vi "FeedbackDecode_20200902.vi"() -> ()   [LabVIEW 2016]
uses:
  FeedbackDecode_DecodeClust.ctl
  FeedbackDecode_MvntClust.ctl
  FeedbackDecode_EncodeClust.ctl
  FeedbackDecode_CogLoadClust.ctl
  <vilib>/Platform/TimedLoop/XDataNode/timing_clust.ctl
  <vilib>/Platform/TimedLoop/XDataNode/nitl_modes.ctl
  <vilib>/Platform/TimedLoop/XDataNode/wakeup.ctl
  <vilib>/DAQmx/write.llb/DAQmx Write (Analog DBL 1Chan 1Samp).vi
  subvi/FeedbackDecode_Globals.vi
  <vilib>/imath/engines/lvmath2/RunTimeEngine/BuiltInFunctions/reshapemx/NIMS_[GM]_reshapemx.vi
  <instcachedir>/0/NIMS_[GM]_reshapemx_500BD31B48F5434EA23B2056DCB44201.lvgen/NIMS_[GM]_reshapemx_500BD31B48F5434EA23B2056DCB44201_005.vi
  <vilib>/imath/engines/lvmath2/RunTimeEngine/BuiltInFunctions/rotate90/NIMS_rotate90.vi
  <instcachedir>/0/NIMS_rotate90_7DC1660D109944E092D2EB6E3185A1B6.lvgen/NIMS_rotate90_7DC1660D109944E092D2EB6E3185A1B6_005.vi
  <vilib>/imath/engines/lvmath2/RunTimeEngine/BuiltInFunctions/reshapemx/NIMS_[GV]_reshapemx.vi
  <instcachedir>/0/NIMS_[GV]_reshapemx_314E456D64644EB191D4916921E89AA6.lvgen/NIMS_[GV]_reshapemx_314E456D64644EB191D4916921E89AA6_001.vi
  <vilib>/imath/engines/lvmath2/RunTimeEngine/ErrorHandling/NIMS_Create Error From Enums.vi
  <vilib>/imath/engines/lvmath2/RunTimeEngine/NodeEndStatement/NIMS_NodeEndStatement_Output.vi
  <instcachedir>/0/NIMS_NodeEndStatement_Output_53EC0D466D134D7ABD903AC30B43404B.lvgen/NIMS_NodeEndStatement_Output_53EC0D466D134D7ABD903AC30B43404B_004.vi
  <vilib>/imath/engines/lvmath2/RunTimeEngine/ErrorHandling/NIMS_Finalize Error.vi
  subvi/FeedbackDecode_VariablesToString_Scalar.vi
  <vilib>/DAQmx/miscellaneous.llb/DAQmx Fill In Error Info.vi
  subvi/FeedbackDecode_VariablesToString_String.vi
  subvi/FeedbackDecode_VariablesToString_Array.vi
  <vilib>/Utility/file.llb/Read Delimited Spreadsheet (string).vi
  <vilib>/Utility/file.llb/Write Delimited Spreadsheet (string).vi
  <vilib>/platform/TimedLoop/XDataNode/XDataNode.xnode
  <vilib>/regexp/Match Regular Expression.xnode
  <vilib>/Platform/TimedLoop/XDataNode/XDNodeRunTimeDep.lvlib
  <resource>/objmgr/daqmx.rc
panel:
  out "CurrMvnt":T1
  in  "Exclude SE":bool
  out "DAQmx?":bool
  out "NumComp":enum16{"1 Computer", "2 Computers"}(ring)
  out "BuildDir":path
  out "PupilTracker":bool
  out "CopySucc":bool
  out "Delete from D drive?":bool
  out "Copy to raid?":bool
  out "Don't save to database?":bool
  out "NextIdx":dbl
  in  "HeatMap Range":cluster{"Min":dbl, "Max":dbl}={"Min"=0.0, "Max"=50.0}
  out "RespRefArray":refnum<vi>[](array[refnum])
  out "VRELabel":T2(ring)
  out "StimTog":bool
  out "SelTog":bool
  out "StimCmd":string
  out "RespStr":string
  out "EvntReg":refnum<event-registration>
  out "MvntEvnt":refnum<user-event>
  out "DataDir":path
  out "PulseStim":bool
  out "BaseCnt3":i64
  out "NIPTime":dbl
  out "ParamsTableLoc":cluster{"Left":i32, "Width":u32}
  out "iTiming":T3
  in  "LVTab":T4(tab)
  out "TrainCnt":dbl
  in  "DecodeClust":T5={"TrainParams"={"Lag"=0.0, "KernelWidth"=0.3, "TargRad"=0.15}, "Kinematics"={"Thumb"=0.0, "Index"=0.0, "Middle"=0.0, "Ring"=0.0, "Little"=0.0, "ThumbInt"=0.0, "IndexInt"=0.0, "RingInt"=0.0, "LittleInt"=0.0, "Wrist"=0.0, "WristYaw"=0.0, "WristRoll"=0.0}, "CtrlButtons"={"AcqTraining"=FALSE, "ApplyBaseline"=FALSE, "ApplyTraining"=FALSE, "LoadTrainFile"=FALSE, "CAR"=FALSE, "NIPSpikes"=FALSE, "AcqBaseline"=FALSE, "Stop"=FALSE, "ResetTrial"=FALSE, "CalDEKA"=FALSE, "HideSphrs"=FALSE, "StartTrials"=FALSE, "AutoPop"=FALSE, "ResetVRE"=FALSE, "StopVRE"=FALSE, "AcqCAR"=FALSE, "ConARD"=FALSE, "DEKARestart"=FALSE, "ConnDEKA"=FALSE}, "CompID"={"LV"={"Name"="PNILABVIEW", "IP"="155.100.90.215"}, "ML"={"Name"="PNIMATLAB", "IP"="155.100.91.231"}}, "KMvntClust"={"KGain"=[[1.0, 1.0, -1.0, 1.0], [1.0, 1.0, -1.0, 1.0], [1.0, 1.0, -1.0, 1.0], [1.0, 1.0, -1.0, 1.0], [1.0, 1.0, -1.0, 1.0], [1.0, 1.0, -1.0, 1.0], [1.0, 1.0, -1.0, 1.0], [1.0, 1.0, -1.0, 1.0], [1.0, 1.0, -1.0, 1.0], [1.0, 1.0, -1.0, 1.0], [1.0, 1.0, -1.0, 1.0], [1.0, 1.0, -1.0, 1.0]], "KMvnts"={"Thumb"=TRUE, "Index"=TRUE, "Middle"=TRUE, "Ring"=TRUE, "Little"=TRUE, "ThumbInt"=TRUE, "IndexInt"=TRUE, "RingInt"=TRUE, "LittleInt"=TRUE, "WristPitch"=TRUE, "WristYaw"=TRUE, "WristRoll"=TRUE}, "KThresh"=[[0.2, 0.2, -1.0, 1.0], [0.2, 0.2, -1.0, 1.0], [0.2, 0.2, -1.0, 1.0], [0.2, 0.2, -1.0, 1.0], [0.2, 0.2, -1.0, 1.0], [0.2, 0.2, -1.0, 1.0], [0.2, 0.2, -1.0, 1.0], [0.2, 0.2, -1.0, 1.0], [0.2, 0.2, -1.0, 1.0], [0.2, 0.2, -1.0, 1.0], [0.2, 0.2, -1.0, 1.0], [0.2, 0.2, -1.0, 1.0]], "CtrlMode"=[enum."Position", enum."Position", enum."Position", enum."Position", enum."Position", enum."Position", enum."Position", enum."Position", enum."Position", enum."Position", enum."Position", enum."Position"], "CtrlSpd"=[1.0, 1.0, 1.0, 1.0, 1.0, 1.0, 1.0, 1.0, 1.0, 1.0, 1.0, 1.0]}, "ClearUEA"=FALSE, "Targets"={"Thumb"=0.0, "Index"=0.0, "Middle"=0.0, "Ring"=0.0, "Little"=0.0, "ThumbInt"=0.0, "IndexInt"=0.0, "RingInt"=0.0, "LittleInt"=0.0, "Wrist"=0.0, "WristYaw"=0.0, "WristRoll"=0.0}, "KUEAArray"=[{"Boolean 1"=FALSE, "Boolean 2"=FALSE, "Boolean 3"=FALSE, "Boolean 4"=FALSE, "Boolean 5"=FALSE, "Boolean 6"=FALSE, "Boolean 7"=FALSE, "Boolean 8"=FALSE, "Boolean 9"=FALSE, "Boolean 10"=FALSE, "Boolean 11"=FALSE, "Boolean 12"=FALSE, "Boolean 13"=FALSE, "Boolean 14"=FALSE, "Boolean 15"=FALSE, "Boolean 16"=FALSE, "Boolean 17"=FALSE, "Boolean 18"=FALSE, "Boolean 19"=FALSE, "Boolean 20"=FALSE, "Boolean 21"=FALSE, "Boolean 22"=FALSE, "Boolean 23"=FALSE, "Boolean 24"=FALSE, "Boolean 25"=FALSE, "Boolean 26"=FALSE, "Boolean 27"=FALSE, "Boolean 28"=FALSE, "Boolean 29"=FALSE, "Boolean 30"=FALSE, "Boolean 31"=FALSE, "Boolean 32"=FALSE, "Boolean 33"=FALSE, "Boolean 34"=FALSE, "Boolean 35"=FALSE, "Boolean 36"=FALSE, "Boolean 37"=FALSE, "Boolean 38"=FALSE, "Boolean 39"=FALSE, "Boolean 40"=FALSE, "Boolean 41"=FALSE, "Boolean 42"=FALSE, "Boolean 43"=FALSE, "Boolean 44"=FALSE, "Boolean 45"=FALSE, "Boolean 46"=FALSE, "Boolean 47"=FALSE, "Boolean 48"=FALSE, "Boolean 49"=FALSE, "Boolean 50"=FALSE, "Boolean 51"=FALSE, "Boolean 52"=FALSE, "Boolean 53"=FALSE, "Boolean 54"=FALSE, "Boolean 55"=FALSE, "Boolean 56"=FALSE, "Boolean 57"=FALSE, "Boolean 58"=FALSE, "Boolean 59"=FALSE, "Boolean 60"=FALSE, "Boolean 61"=FALSE, "Boolean 62"=FALSE, "Boolean 63"=FALSE, "Boolean 64"=FALSE, "Boolean 65"=FALSE, "Boolean 66"=FALSE, "Boolean 67"=FALSE, "Boolean 68"=FALSE, "Boolean 69"=FALSE, "Boolean 70"=FALSE, "Boolean 71"=FALSE, "Boolean 72"=FALSE, "Boolean 73"=FALSE, "Boolean 74"=FALSE, "Boolean 75"=FALSE, "Boolean 76"=FALSE, "Boolean 77"=FALSE, "Boolean 78"=FALSE, "Boolean 79"=FALSE, "Boolean 80"=FALSE, "Boolean 81"=FALSE, "Boolean 82"=FALSE, "Boolean 83"=FALSE, "Boolean 84"=FALSE, "Boolean 85"=FALSE, "Boolean 86"=FALSE, "Boolean 87"=FALSE, "Boolean 88"=FALSE, "Boolean 89"=FALSE, "Boolean 90"=FALSE, "Boolean 91"=FALSE, "Boolean 92"=FALSE, "Boolean 93"=FALSE, "Boolean 94"=FALSE, "Boolean 95"=FALSE, "Boolean 96"=FALSE, "Boolean 97"=FALSE, "Boolean 98"=FALSE, "Boolean 99"=FALSE, "Boolean 100"=FALSE}, {"Boolean 1"=FALSE, "Boolean 2"=FALSE, "Boolean 3"=FALSE, "Boolean 4"=FALSE, "Boolean 5"=FALSE, "Boolean 6"=FALSE, "Boolean 7"=FALSE, "Boolean 8"=FALSE, "Boolean 9"=FALSE, "Boolean 10"=FALSE, "Boolean 11"=FALSE, "Boolean 12"=FALSE, "Boolean 13"=FALSE, "Boolean 14"=FALSE, "Boolean 15"=FALSE, "Boolean 16"=FALSE, "Boolean 17"=FALSE, "Boolean 18"=FALSE, "Boolean 19"=FALSE, "Boolean 20"=FALSE, "Boolean 21"=FALSE, "Boolean 22"=FALSE, "Boolean 23"=FALSE, "Boolean 24"=FALSE, "Boolean 25"=FALSE, "Boolean 26"=FALSE, "Boolean 27"=FALSE, "Boolean 28"=FALSE, "Boolean 29"=FALSE, "Boolean 30"=FALSE, "Boolean 31"=FALSE, "Boolean 32"=FALSE, "Boolean 33"=FALSE, "Boolean 34"=FALSE, "Boolean 35"=FALSE, "Boolean 36"=FALSE, "Boolean 37"=FALSE, "Boolean 38"=FALSE, "Boolean 39"=FALSE, "Boolean 40"=FALSE, "Boolean 41"=FALSE, "Boolean 42"=FALSE, "Boolean 43"=FALSE, "Boolean 44"=FALSE, "Boolean 45"=FALSE, "Boolean 46"=FALSE, "Boolean 47"=FALSE, "Boolean 48"=FALSE, "Boolean 49"=FALSE, "Boolean 50"=FALSE, "Boolean 51"=FALSE, "Boolean 52"=FALSE, "Boolean 53"=FALSE, "Boolean 54"=FALSE, "Boolean 55"=FALSE, "Boolean 56"=FALSE, "Boolean 57"=FALSE, "Boolean 58"=FALSE, "Boolean 59"=FALSE, "Boolean 60"=FALSE, "Boolean 61"=FALSE, "Boolean 62"=FALSE, "Boolean 63"=FALSE, "Boolean 64"=FALSE, "Boolean 65"=FALSE, "Boolean 66"=FALSE, "Boolean 67"=FALSE, "Boolean 68"=FALSE, "Boolean 69"=FALSE, "Boolean 70"=FALSE, "Boolean 71"=FALSE, "Boolean 72"=FALSE, "Boolean 73"=FALSE, "Boolean 74"=FALSE, "Boolean 75"=FALSE, "Boolean 76"=FALSE, "Boolean 77"=FALSE, "Boolean 78"=FALSE, "Boolean 79"=FALSE, "Boolean 80"=FALSE, "Boolean 81"=FALSE, "Boolean 82"=FALSE, "Boolean 83"=FALSE, "Boolean 84"=FALSE, "Boolean 85"=FALSE, "Boolean 86"=FALSE, "Boolean 87"=FALSE, "Boolean 88"=FALSE, "Boolean 89"=FALSE, "Boolean 90"=FALSE, "Boolean 91"=FALSE, "Boolean 92"=FALSE, "Boolean 93"=FALSE, "Boolean 94"=FALSE, "Boolean 95"=FALSE, "Boolean 96"=FALSE, "Boolean 97"=FALSE, "Boolean 98"=FALSE, "Boolean 99"=FALSE, "Boolean 100"=FALSE}], "ReTrain"=FALSE, "TargDist"=[0.0, 0.0, 0.0, 0.0, 0.0, 0.0], "State"=enum."Initialize", "KalmanType"=enum."Mean", "EventStr"="", "SelElect"=1.0, "KinSrc"=enum."Off", "HoverElect"=1.0, "RasterWin"=15.0, "WfCnt"=50.0, "ClearWfs"=FALSE, "ApplyThresh"=FALSE, "ThreshVal"=-5.0, "ThreshMode"=enum."RMS Auto", "DataFolder"="00000000-000000", "ClearEMG"=FALSE, "KEMGClust"={"Boolean 92"=FALSE, "Boolean 82"=FALSE, "Boolean 72"=FALSE, "Boolean 62"=FALSE, "Boolean 52"=FALSE, "Boolean 42"=FALSE, "Boolean 32"=FALSE, "Boolean 22"=FALSE, "Boolean 12"=FALSE, "Boolean 2"=FALSE, "Boolean 93"=FALSE, "Boolean 83"=FALSE, "Boolean 73"=FALSE, "Boolean 63"=FALSE, "Boolean 53"=FALSE, "Boolean 43"=FALSE, "Boolean 33"=FALSE, "Boolean 23"=FALSE, "Boolean 13"=FALSE, "Boolean 3"=FALSE, "Boolean 94"=FALSE, "Boolean 84"=FALSE, "Boolean 74"=FALSE, "Boolean 64"=FALSE, "Boolean 54"=FALSE, "Boolean 44"=FALSE, "Boolean 34"=FALSE, "Boolean 24"=FALSE, "Boolean 14"=FALSE, "Boolean 4"=FALSE, "Boolean 95"=FALSE, "Boolean 85"=FALSE, "Boolean 75"=FALSE, "Boolean 65"=FALSE, "Boolean 55"=FALSE, "Boolean 45"=FALSE, "Boolean 35"=FALSE, "Boolean 25"=FALSE, "Boolean 15"=FALSE, "Boolean 5"=FALSE, "Boolean 96"=FALSE, "Boolean 86"=FALSE, "Boolean 76"=FALSE, "Boolean 66"=FALSE, "Boolean 56"=FALSE, "Boolean 46"=FALSE, "Boolean 36"=FALSE, "Boolean 26"=FALSE, "Boolean 16"=FALSE, "Boolean 6"=FALSE, "Boolean 97"=FALSE, "Boolean 87"=FALSE, "Boolean 77"=FALSE, "Boolean 67"=FALSE, "Boolean 57"=FALSE, "Boolean 47"=FALSE, "Boolean 37"=FALSE, "Boolean 27"=FALSE, "Boolean 17"=FALSE, "Boolean 7"=FALSE, "Boolean 98"=FALSE, "Boolean 88"=FALSE, "Boolean 78"=FALSE, "Boolean 68"=FALSE, "Boolean 58"=FALSE, "Boolean 48"=FALSE, "Boolean 38"=FALSE, "Boolean 28"=FALSE, "Boolean 18"=FALSE, "Boolean 8"=FALSE, "Boolean 99"=FALSE, "Boolean 89"=FALSE, "Boolean 79"=FALSE, "Boolean 69"=FALSE, "Boolean 59"=FALSE, "Boolean 49"=FALSE, "Boolean 39"=FALSE, "Boolean 29"=FALSE, "Boolean 19"=FALSE, "Boolean 9"=FALSE}, "EvntFlag"=FALSE, "FillUEA"=FALSE, "FillEMG"=FALSE, "FillMvnts"=FALSE, "BadUEAElects"=[], "KEMGExtra"=[], "AllPairs"=TRUE, "AutoThresh"=0.4, "BadEMGChans"=[], "LinkedDOF"="{}", "AutoPopType"=enum."Gram", "CARType"=enum."Standard", "*Map"=enum."pNeural/pEMG", "GainFill"=1.0, "ThreshFill"=0.2, "TestType"=enum."MSMS", "Outcome"=enum."---", "TrialCnt"=[[0.0, 0.0, 0.0, 0.0, 0.0, 0.0, 0.0, 0.0, 0.0, 0.0, 0.0, 0.0], [0.0, 0.0, 0.0, 0.0, 0.0, 0.0, 0.0, 0.0, 0.0, 0.0, 0.0, 0.0]], "ClearTrials"=FALSE, "Log10"=FALSE, "KDFFile"="", "LimitExt"=FALSE, "*Prosthesis"=enum."MaleRight", "StartML"=TRUE, "StartMLAux"=TRUE, "StartRec"=TRUE, "DynaThr"=FALSE, "ModeFill"=enum."Position", "SpdFill"=1.0, "DEKAMode"=enum."Position", "FreeParam"=1.0, "GoalNoise"=0.0, "Load NN"=FALSE, "ExportTrain"=FALSE, "NumComp"=enum."2 Computers", "DataDir"="00000000-000000", "BuildDir"="00000000-000000", "LatchingFilter"=FALSE, "Trigger"=FALSE} {"SpdFill" min=0.0 max=10.0 step=0.1; "RasterWin" min=1.0 max=30.0 step=1.0; "ThreshFill" min=0.0 max=10.0 step=0.01; "GainFill" min=0.0 max=10.0 step=0.1; "AutoThresh" min=0.0 max=1.0; "Targets"."LittleInt" min=0.0 max=1.0 step=0.01; "Targets"."WristRoll" min=0.0 max=1.0 step=0.01; "Targets"."WristYaw" min=0.0 max=1.0 step=0.01; "Targets"."Wrist" min=0.0 max=1.0 step=0.01; "Targets"."Little" min=0.0 max=1.0 step=0.01; "Targets"."Thumb" min=0.0 max=1.0 step=0.01; "Targets"."RingInt" min=0.0 max=1.0 step=0.01; "Targets"."IndexInt" min=0.0 max=1.0 step=0.01; "Targets"."ThumbInt" min=0.0 max=1.0 step=0.01; "Targets"."Ring" min=0.0 max=1.0 step=0.01; "Targets"."Middle" min=0.0 max=1.0 step=0.01; "Targets"."Index" min=0.0 max=1.0 step=0.01; "KMvntClust"."CtrlSpd" min=0 max=10; "KMvntClust"."KThresh" min=0 max=1; "KMvntClust"."KGain" min=0; "Kinematics"."LittleInt" min=0.0 max=1.0 step=0.01; "Kinematics"."WristRoll" min=0.0 max=1.0 step=0.01; "Kinematics"."WristYaw" min=0.0 max=1.0 step=0.01; "Kinematics"."Wrist" min=0.0 max=1.0 step=0.01; "Kinematics"."Little" min=0.0 max=1.0 step=0.01; "Kinematics"."Thumb" min=0.0 max=1.0 step=0.01; "Kinematics"."RingInt" min=0.0 max=1.0 step=0.01; "Kinematics"."IndexInt" min=0.0 max=1.0 step=0.01; "Kinematics"."ThumbInt" min=0.0 max=1.0 step=0.01; "Kinematics"."Ring" min=0.0 max=1.0 step=0.01; "Kinematics"."Middle" min=0.0 max=1.0 step=0.01; "Kinematics"."Index" min=0.0 max=1.0 step=0.01; "TrainParams"."TargRad" step=0.05 format="%#.2g"; "TrainParams"."KernelWidth" step=0.05 format="%#.2g"}
  in  "Timing":T3={"Dur"={"ASD"=1000.0, "ARD"=5000.0, "ART"=5000.0, "ETD"=500.0}, "Rnd"={"ASDR"=0.0, "ARDR"=0.0, "ARTR"=0.0, "ETDR"=0.0}, "Act"={"ASDA"=0.0, "ARDA"=0.0, "ARTA"=0.0, "ETDA"=0.0}}
  in  "MvntBuilder":T6={"MvntType"={"Thumb"=enum."False", "Index"=enum."False", "Middle"=enum."False", "Ring"=enum."False", "Little"=enum."False", "ThumbInt"=enum."False", "IndexInt"=enum."False", "RingInt"=enum."False", "LittleInt"=enum."False", "WristPitch"=enum."False", "WristYaw"=enum."False", "WristRoll"=enum."False"}, "MvntParams"={"Amp"=1.0, "Delay"=0.0, "Rise"=0.7, "Hold"=3.0}, "MvntList"=[{"MvntMat"=[[0.0, 0.0, 0.0, 0.0], [0.0, 0.0, 0.0, 0.0], [0.0, 0.0, 0.0, 0.0], [0.0, 0.0, 0.0, 0.0], [0.0, 0.0, 0.0, 0.0], [0.0, 0.0, 0.0, 0.0], [0.0, 0.0, 0.0, 0.0], [0.0, 0.0, 0.0, 0.0], [0.0, 0.0, 0.0, 0.0], [0.0, 0.0, 0.0, 0.0], [0.0, 0.0, 0.0, 0.0], [0.0, 0.0, 0.0, 0.0]], "MvntName"="", "Tracking"=enum."False", "Radius"=0.15}], "Set"=FALSE, "Clear"=FALSE, "Load"=FALSE, "Mode"=enum."Block", "NTrials"=10.0, "TargParams"={"Gain"=1.0, "Radius"=0.15, "Acc"=0.8}, "Save"=FALSE, "PercTrials"=0.0} {"PercTrials" format="%#_2g"; "NTrials" min=1.0 max=100.0 step=1.0; "MvntList"."Radius" min=0.0 max=1.0 step=0.01; "TargParams"."Acc" min=0.0 max=1.0 step=0.01; "TargParams"."Radius" min=0.0 max=1.0 step=0.01; "TargParams"."Gain" min=-1.0 max=1.0 step=0.01; "MvntParams"."Hold" min=0.0 step=0.1; "MvntParams"."Rise" min=0.0 step=0.1; "MvntParams"."Delay" min=0.0 step=0.1; "MvntParams"."Amp" min=-1.0 max=1.0 step=0.1}
  in  "ManualClust":T7 {"WristRoll" scale=-1.0..1.0; "WristYaw" scale=-1.0..1.0; "WristPitch" scale=-1.0..1.0; "LittleInt" scale=-1.0..1.0; "RingInt" scale=-1.0..1.0; "IndexInt" scale=-1.0..1.0; "ThumbInt" scale=-1.0..1.0; "Little" scale=-1.0..1.0; "Ring" scale=-1.0..1.0; "Middle" scale=-1.0..1.0; "Index" scale=-1.0..1.0; "Thumb" scale=-1.0..1.0}
  in  "ManualDOF":T8
  in  "EncodeClust":T9={"ParamsTable"=[], "Sel"=[], "Stim"=FALSE, "StimMode"=enum."Off", "StimStep"=[enum."1uA", enum."1uA", enum."Off"], "Jitter"=FALSE, "Pulse"=FALSE, "BFreq"=0.0, "BAmp"=0.0, "UEAArray"=[{"Boolean 1"=FALSE, "Boolean 2"=FALSE, "Boolean 3"=FALSE, "Boolean 4"=FALSE, "Boolean 5"=FALSE, "Boolean 6"=FALSE, "Boolean 7"=FALSE, "Boolean 8"=FALSE, "Boolean 9"=FALSE, "Boolean 10"=FALSE, "Boolean 11"=FALSE, "Boolean 12"=FALSE, "Boolean 13"=FALSE, "Boolean 14"=FALSE, "Boolean 15"=FALSE, "Boolean 16"=FALSE, "Boolean 17"=FALSE, "Boolean 18"=FALSE, "Boolean 19"=FALSE, "Boolean 20"=FALSE, "Boolean 21"=FALSE, "Boolean 22"=FALSE, "Boolean 23"=FALSE, "Boolean 24"=FALSE, "Boolean 25"=FALSE, "Boolean 26"=FALSE, "Boolean 27"=FALSE, "Boolean 28"=FALSE, "Boolean 29"=FALSE, "Boolean 30"=FALSE, "Boolean 31"=FALSE, "Boolean 32"=FALSE, "Boolean 33"=FALSE, "Boolean 34"=FALSE, "Boolean 35"=FALSE, "Boolean 36"=FALSE, "Boolean 37"=FALSE, "Boolean 38"=FALSE, "Boolean 39"=FALSE, "Boolean 40"=FALSE, "Boolean 41"=FALSE, "Boolean 42"=FALSE, "Boolean 43"=FALSE, "Boolean 44"=FALSE, "Boolean 45"=FALSE, "Boolean 46"=FALSE, "Boolean 47"=FALSE, "Boolean 48"=FALSE, "Boolean 49"=FALSE, "Boolean 50"=FALSE, "Boolean 51"=FALSE, "Boolean 52"=FALSE, "Boolean 53"=FALSE, "Boolean 54"=FALSE, "Boolean 55"=FALSE, "Boolean 56"=FALSE, "Boolean 57"=FALSE, "Boolean 58"=FALSE, "Boolean 59"=FALSE, "Boolean 60"=FALSE, "Boolean 61"=FALSE, "Boolean 62"=FALSE, "Boolean 63"=FALSE, "Boolean 64"=FALSE, "Boolean 65"=FALSE, "Boolean 66"=FALSE, "Boolean 67"=FALSE, "Boolean 68"=FALSE, "Boolean 69"=FALSE, "Boolean 70"=FALSE, "Boolean 71"=FALSE, "Boolean 72"=FALSE, "Boolean 73"=FALSE, "Boolean 74"=FALSE, "Boolean 75"=FALSE, "Boolean 76"=FALSE, "Boolean 77"=FALSE, "Boolean 78"=FALSE, "Boolean 79"=FALSE, "Boolean 80"=FALSE, "Boolean 81"=FALSE, "Boolean 82"=FALSE, "Boolean 83"=FALSE, "Boolean 84"=FALSE, "Boolean 85"=FALSE, "Boolean 86"=FALSE, "Boolean 87"=FALSE, "Boolean 88"=FALSE, "Boolean 89"=FALSE, "Boolean 90"=FALSE, "Boolean 91"=FALSE, "Boolean 92"=FALSE, "Boolean 93"=FALSE, "Boolean 94"=FALSE, "Boolean 95"=FALSE, "Boolean 96"=FALSE, "Boolean 97"=FALSE, "Boolean 98"=FALSE, "Boolean 99"=FALSE, "Boolean 100"=FALSE}, {"Boolean 1"=FALSE, "Boolean 2"=FALSE, "Boolean 3"=FALSE, "Boolean 4"=FALSE, "Boolean 5"=FALSE, "Boolean 6"=FALSE, "Boolean 7"=FALSE, "Boolean 8"=FALSE, "Boolean 9"=FALSE, "Boolean 10"=FALSE, "Boolean 11"=FALSE, "Boolean 12"=FALSE, "Boolean 13"=FALSE, "Boolean 14"=FALSE, "Boolean 15"=FALSE, "Boolean 16"=FALSE, "Boolean 17"=FALSE, "Boolean 18"=FALSE, "Boolean 19"=FALSE, "Boolean 20"=FALSE, "Boolean 21"=FALSE, "Boolean 22"=FALSE, "Boolean 23"=FALSE, "Boolean 24"=FALSE, "Boolean 25"=FALSE, "Boolean 26"=FALSE, "Boolean 27"=FALSE, "Boolean 28"=FALSE, "Boolean 29"=FALSE, "Boolean 30"=FALSE, "Boolean 31"=FALSE, "Boolean 32"=FALSE, "Boolean 33"=FALSE, "Boolean 34"=FALSE, "Boolean 35"=FALSE, "Boolean 36"=FALSE, "Boolean 37"=FALSE, "Boolean 38"=FALSE, "Boolean 39"=FALSE, "Boolean 40"=FALSE, "Boolean 41"=FALSE, "Boolean 42"=FALSE, "Boolean 43"=FALSE, "Boolean 44"=FALSE, "Boolean 45"=FALSE, "Boolean 46"=FALSE, "Boolean 47"=FALSE, "Boolean 48"=FALSE, "Boolean 49"=FALSE, "Boolean 50"=FALSE, "Boolean 51"=FALSE, "Boolean 52"=FALSE, "Boolean 53"=FALSE, "Boolean 54"=FALSE, "Boolean 55"=FALSE, "Boolean 56"=FALSE, "Boolean 57"=FALSE, "Boolean 58"=FALSE, "Boolean 59"=FALSE, "Boolean 60"=FALSE, "Boolean 61"=FALSE, "Boolean 62"=FALSE, "Boolean 63"=FALSE, "Boolean 64"=FALSE, "Boolean 65"=FALSE, "Boolean 66"=FALSE, "Boolean 67"=FALSE, "Boolean 68"=FALSE, "Boolean 69"=FALSE, "Boolean 70"=FALSE, "Boolean 71"=FALSE, "Boolean 72"=FALSE, "Boolean 73"=FALSE, "Boolean 74"=FALSE, "Boolean 75"=FALSE, "Boolean 76"=FALSE, "Boolean 77"=FALSE, "Boolean 78"=FALSE, "Boolean 79"=FALSE, "Boolean 80"=FALSE, "Boolean 81"=FALSE, "Boolean 82"=FALSE, "Boolean 83"=FALSE, "Boolean 84"=FALSE, "Boolean 85"=FALSE, "Boolean 86"=FALSE, "Boolean 87"=FALSE, "Boolean 88"=FALSE, "Boolean 89"=FALSE, "Boolean 90"=FALSE, "Boolean 91"=FALSE, "Boolean 92"=FALSE, "Boolean 93"=FALSE, "Boolean 94"=FALSE, "Boolean 95"=FALSE, "Boolean 96"=FALSE, "Boolean 97"=FALSE, "Boolean 98"=FALSE, "Boolean 99"=FALSE, "Boolean 100"=FALSE}], "AdjClust"={"Add"=FALSE, "Sub"=FALSE, "Val"=[1.0, 100.0, 10.0, 500.0, 0.2], "B"=[FALSE, FALSE, FALSE, FALSE, FALSE], "Inc+"=["x+1", "x+1", "x+10", "x+10", "x+0.1"], "Set"=FALSE, "LoadTable"=FALSE, "SaveTable"=FALSE, "ClearTable"=FALSE, "DeleteSel"=FALSE, "Inc-"=["x-1", "x-1", "x-10", "x-10", "x-0.1"]}, "PresetTable"=[], "SelPreset"=[], "SortClust"={"Region"=FALSE, "Receptor"=FALSE, "Electrode"=FALSE, "Min Amp"=FALSE, "Max Amp"=FALSE, "Min Freq"=FALSE, "Max Freq"=FALSE, "Duration"=FALSE}, "SelSort"={"Sel"=FALSE}, "PresetClust"={"Load"=FALSE, "Clear"=FALSE, "Save"=FALSE, "Del"=FALSE}, "RespClust"={"RespType"=enum."Sensor Map", "OpenResp"=FALSE}, "AmpLimit"=100.0, "FreqLimit"=500.0, "DurLimit"=0.2, "Wait Period"=0.5, "Train Period"=0.5} {"Train Period" min=0.0 max=100.0 step=0.1; "Wait Period" min=0.0 max=100.0 step=0.1; "DurLimit" min=0.0 max=1.0 step=0.01; "FreqLimit" min=0.0 max=500.0 step=1.0; "AmpLimit" min=0.0 max=100.0 step=1.0; "BAmp" min=0.0 max=100.0 step=1.0; "BFreq" min=0.0 max=100.0 step=1.0}
  in  "Sensor Tab Control":enum32{"DEKA", "Analog", "TASKA"}(tab)
  out "DekaSensors":waveform(dbl)[](graph)
  out "StimWfGraph":dbl[](graph)
  in  "Stim Thresholds":dbl[](array[numeric])=[0.0, 0.0, 0.0, 0.0, 0.0, 0.0, 0.0, 0.0, 0.0, 0.0, 0.0, 0.0, 0.0]
  in  "DekaSensorBreakThreshold":dbl[](array[numeric])=[40.0, 40.0, 40.0, 40.0, 40.0, 40.0, 40.0, 40.0, 40.0, 40.0, 40.0, 40.0, 40.0]
  out "AnlgPlot":waveform(dbl)[](graph)=[{"t0"=timestamp(27834 s since 1904-01-01), "dt"=1.0, "Y"=[2.75375102500714]}, {"t0"=timestamp(27834 s since 1904-01-01), "dt"=1.0, "Y"=[2.3160330296785294]}, {"t0"=timestamp(27834 s since 1904-01-01), "dt"=1.0, "Y"=[1.270290647354958]}, {"t0"=timestamp(27834 s since 1904-01-01), "dt"=1.0, "Y"=[1.3014283460420921]}]
  in  "OffSet":dbl
  in  "LoadCyberGlove":bool
  in  "TASKARestPositions":string="Rest Positions"
  in  "ThumbIntSet":dbl caption="ThumbInt" min=0.0 max=1.0
  in  "ThumbSet":dbl caption="Thumb" min=0.0 max=1.0
  in  "PinkySet":dbl caption="Pinky" min=0.0 max=1.0
  in  "RingSet":dbl caption="Ring" min=0.0 max=1.0
  in  "MiddleSet":dbl caption="Middle" min=0.0 max=1.0
  in  "IndexSet":dbl caption="Index" min=0.0 max=1.0
  in  "CalibrateTASKA":bool
  in  "Beta Mode":string(combo)="Fixed"
  in  "Computer Goal":string(combo)="Close"
  out "TASKA Pressure":waveform(dbl)[](graph)=[{"t0"=timestamp(87262 s since 1904-01-01), "dt"=1.0, "Y"=[0.0]}, {"t0"=timestamp(87262 s since 1904-01-01), "dt"=1.0, "Y"=[0.0]}, {"t0"=timestamp(87262 s since 1904-01-01), "dt"=1.0, "Y"=[0.0]}]
  out "TASKA IR":waveform(dbl)[](graph)=[{"t0"=timestamp(87262 s since 1904-01-01), "dt"=1.0, "Y"=[4.0]}, {"t0"=timestamp(87262 s since 1904-01-01), "dt"=1.0, "Y"=[0.0]}, {"t0"=timestamp(87262 s since 1904-01-01), "dt"=1.0, "Y"=[0.0]}]
  in  "TASKA Shared Control":bool
  in  "TASKASharedControlBeta":dbl caption="Beta" min=0.0 max=1.0
  in  "ThumbShare":bool
  in  "IndexShare":bool
  in  "RingShare":bool
  in  "MiddleShare":bool
  in  "Reset Calibration":bool
  in  "TASKASharedControlIncrememnt":dbl caption="Inc." min=0.0 max=1.0
  in  "TASKA Timer":bool
  in  "TASKA Reset Break":bool
  in  "TASKA Reset Success":bool
  out "WAVChart":dbl[](graph)=[0.01885986328125, 0.02471923828125, 0.026458740234375, 0.019622802734375, 0.015625, 0.016571044921875, 0.017852783203125, 0.016937255859375, 0.02349853515625, 0.0262451171875, 0.021697998046875, 0.01995849609375, 0.013427734375, 0.008819580078125, 0.013916015625, 0.016693115234375, 0.0172119140625, 0.023468017578125, 0.0235595703125, 0.018890380859375, 0.022369384765625, 0.022003173828125, 0.019378662109375, 0.017578125, 0.0115966796875, 0.011688232421875, 0.011016845703125, 0.007659912109375, 0.012359619140625, 0.015167236328125, 0.010162353515625, 0.00787353515625, 0.010009765625, 0.01434326171875, 0.018524169921875, 0.019012451171875, 0.019317626953125, 0.019500732421875, 0.021514892578125, 0.021514892578125, 0.0233154296875, 0.02276611328125, 0.0174560546875, 0.018585205078125, 0.019439697265625, 0.01959228515625, 0.0185546875, 0.015594482421875, 0.01593017578125, 0.0162353515625, 0.013427734375, 0.01519775390625, 0.005340576171875, 0.008026123046875, 0.00811767578125, 0.004669189453125, 0.008148193359375, 0.00384521484375, 0.007598876953125, 0.007354736328125, 0.009735107421875, 0.01580810546875, 0.01385498046875, 0.014923095703125, 0.00830078125, 0.005096435546875, 0.008941650390625, 0.01416015625, 0.01220703125, 0.0140380859375, 0.01275634765625, 0.006439208984375, 0.007049560546875, 0.006134033203125, -0.000457763671875, 0.003326416015625, 0.0081787109375, 0.009124755859375, 0.013458251953125, 0.014007568359375, 0.014312744140625, 0.006011962890625, 0.00238037109375, 0.010284423828125, 0.011962890625, 0.009857177734375, 0.00909423828125, 0.016448974609375, 0.01885986328125, 0.01190185546875, 0.010955810546875, 0.01019287109375, 0.00152587890625, 0.00762939453125, 0.008270263671875, 0.00604248046875, 0.010589599609375, 0.0037841796875, 0.0050048828125, 0.007080078125, 0.004669189453125, 0.0064697265625, 0.01068115234375, 0.009521484375, 0.002532958984375, -0.000518798828125, 0.005035400390625, 0.0042724609375, 0.00164794921875, 0.0001220703125, -0.002716064453125, -0.00164794921875, -0.007232666015625, -0.01153564453125, -0.005889892578125, -0.00341796875, -0.008514404296875, -0.007415771484375, -0.00726318359375, -0.007781982421875, -0.009918212890625, -0.010772705078125, -0.00628662109375, -0.001373291015625, -0.0008544921875, -0.003997802734375, 0.003021240234375, 0.003082275390625, 0.000640869140625, 0.00250244140625, 0.002960205078125, 0.00115966796875, 0.000579833984375, -0.002166748046875, -0.00115966796875, -0.006591796875, -0.0128173828125, -0.013275146484375, -0.0157470703125, -0.016204833984375, -0.013885498046875, -0.01531982421875, -0.00897216796875, -0.00762939453125, -0.00738525390625, -0.00311279296875, -0.002166748046875, 0.000244140625, -0.003509521484375, -0.003662109375, 0.001220703125, 0.001251220703125, 0.0001220703125, -0.003692626953125, -0.003997802734375, -0.004364013671875, -9.1552734375e-05, 0.00341796875, 0.000457763671875, -0.000274658203125, -0.0006103515625, 0.00543212890625, 0.001312255859375, 0.003662109375, 0.009765625, 0.004852294921875, 0.003997802734375, 0.00189208984375, -0.000213623046875, -0.006500244140625, -0.006744384765625, -0.0120849609375, -0.012359619140625, -0.003631591796875, -0.005645751953125, -0.0028076171875, 0.00286865234375, -0.00311279296875, -0.005279541015625, 0.001922607421875, -0.003753662109375, -0.000335693359375, -0.00299072265625, 0.001556396484375, 0.00299072265625, 0.006317138671875, 0.006622314453125, -0.003692626953125, -0.007110595703125, 0.001190185546875, -0.002288818359375, 0.00030517578125, 0.007720947265625, 0.003692626953125, 0.006011962890625, 0.007904052734375, 0.0115966796875, 0.01513671875, 0.00421142578125, 0.00299072265625, 0.002532958984375, 0.0009765625, 0.0018310546875, 0.001556396484375, 0.00640869140625, 0.008148193359375, 0.011962890625, 0.01416015625, 0.01055908203125, 0.0126953125, 0.006500244140625, 0.00958251953125, 0.009613037109375, 0.00921630859375, 0.007049560546875, 0.00927734375, 0.011871337890625, 0.015655517578125, 0.0146484375, 0.011627197265625, 0.0162353515625, 0.007965087890625, 0.00146484375, 0.004425048828125, 0.007415771484375, 0.007598876953125, 0.011810302734375, 0.01324462890625, 0.016357421875, 0.0126953125, 0.012451171875, 0.01763916015625, 0.0196533203125, 0.019775390625, 0.021453857421875, 0.025848388671875, 0.023468017578125, 0.01934814453125, 0.019073486328125, 0.020355224609375, 0.021270751953125, 0.024139404296875, 0.02545166015625, 0.0255126953125, 0.027862548828125, 0.027435302734375, 0.030487060546875, 0.029052734375, 0.032196044921875, 0.030120849609375, 0.035552978515625, 0.026611328125, 0.025787353515625, 0.030303955078125, 0.021270751953125, 0.027099609375, 0.032379150390625, 0.03143310546875, 0.02508544921875, 0.03118896484375, 0.029510498046875, 0.0311279296875, 0.03460693359375, 0.0340576171875, 0.027435302734375, 0.03076171875, 0.031707763671875, 0.029815673828125, 0.0341796875, 0.039337158203125, 0.0396728515625, 0.039459228515625, 0.031463623046875, 0.025482177734375, 0.03057861328125, 0.031707763671875, 0.03253173828125, 0.035308837890625, 0.0355224609375, 0.035369873046875, 0.02996826171875, 0.0267333984375, 0.025665283203125, 0.024688720703125, 0.029754638671875, 0.023681640625, 0.02490234375, 0.026458740234375, 0.025726318359375, 0.03436279296875, 0.028411865234375, 0.0225830078125, 0.02349853515625, 0.021270751953125, 0.02691650390625, 0.02520751953125, 0.023101806640625, 0.020782470703125, 0.0198974609375, 0.024200439453125, 0.021148681640625, 0.023406982421875, 0.028289794921875, 0.02862548828125, 0.03240966796875, 0.025634765625, 0.030120849609375, 0.029998779296875, 0.02752685546875, 0.033660888671875, 0.028167724609375, 0.032073974609375, 0.033233642578125, 0.02862548828125, 0.029876708984375, 0.02667236328125, 0.02392578125, 0.02764892578125, 0.026275634765625, 0.023468017578125, 0.031158447265625, 0.0306396484375, 0.022125244140625, 0.022430419921875, 0.025054931640625, 0.02337646484375, 0.025299072265625, 0.02777099609375, 0.03326416015625, 0.02777099609375, 0.025390625, 0.028778076171875, 0.02239990234375, 0.01837158203125, 0.021148681640625, 0.021514892578125, 0.018218994140625, 0.01593017578125, 0.017547607421875, 0.018524169921875, 0.01739501953125, 0.01922607421875, 0.016632080078125, 0.010772705078125, 0.013519287109375, 0.011383056640625, 0.013671875, 0.017242431640625, 0.021636962890625, 0.01922607421875, 0.01593017578125, 0.016571044921875, 0.015777587890625, 0.016693115234375, 0.011260986328125, 0.005828857421875, 0.0068359375, 0.001739501953125, 0.00518798828125, 0.006591796875, 0.00286865234375, 0.015289306640625, 0.011383056640625, 0.01031494140625, 0.00927734375, 0.009307861328125, 0.011199951171875, 0.010894775390625, 0.006927490234375, 0.0115966796875, 0.004638671875, 0.004425048828125, 0.003631591796875, 0.007659912109375, 0.0086669921875, 0.00616455078125, 0.003509521484375, -0.000518798828125, 0.0001220703125, -0.001708984375, -0.0015869140625, 0.002349853515625, 0.0089111328125, 0.007171630859375, 0.0072021484375, 0.004791259765625, 0.00341796875, 0.001068115234375, 0.00341796875, 0.00445556640625, 0.008056640625, 0.009246826171875, 0.011077880859375, 0.006195068359375, 0.005340576171875, 0.00244140625, 0.006561279296875, 0.016021728515625, 0.011322021484375, 0.0079345703125, 0.006622314453125, 0.01080322265625, 0.009796142578125, 0.0028076171875, 0.00439453125, 0.00048828125, 0.0052490234375, 0.0025634765625, 0.00396728515625, 0.0057373046875, 0.00860595703125, 0.00701904296875, 0.0020751953125, -0.00189208984375, -0.001861572265625, 0.00091552734375, -0.00762939453125, -0.0074462890625, -0.0054931640625, 0.0010986328125, 0.00421142578125, 0.001800537109375, 0.007232666015625, -0.001190185546875, 9.1552734375e-05, -0.0078125, -0.010833740234375, -0.0068359375, -0.0054931640625, -0.004791259765625, -0.011016845703125, -0.009765625, -0.007720947265625, -0.00384521484375, -0.011260986328125, -0.00848388671875, -0.000152587890625, -0.00030517578125, -0.00177001953125, -0.0052490234375, -0.00994873046875, -0.001617431640625, -0.00567626953125, -0.008209228515625, -0.004638671875, -0.0057373046875, -0.0067138671875, -0.01080322265625, -0.008544921875, -0.0120849609375, -0.009857177734375, -0.01409912109375, -0.0184326171875, -0.022003173828125, -0.023101806640625, -0.02197265625, -0.021942138671875, -0.018035888671875, -0.016632080078125, -0.025726318359375, -0.032623291015625, -0.02557373046875, -0.03179931640625, -0.020660400390625, -0.017578125, -0.01641845703125, -0.017852783203125, -0.02423095703125, -0.030609130859375, -0.03009033203125, -0.027862548828125, -0.031646728515625, -0.03076171875, -0.0225830078125, -0.015472412109375, -0.018341064453125, -0.02520751953125, -0.032958984375, -0.034759521484375, -0.034637451171875, -0.033233642578125, -0.031768798828125, -0.025238037109375, -0.02752685546875, -0.03057861328125, -0.0286865234375, -0.03204345703125, -0.02850341796875, -0.020965576171875, -0.022735595703125, -0.02435302734375, -0.024383544921875, -0.02496337890625, -0.01910400390625, -0.0230712890625, -0.0225830078125, -0.02435302734375, -0.027984619140625, -0.027740478515625, -0.026153564453125, -0.03021240234375, -0.030792236328125, -0.0277099609375, -0.0250244140625, -0.02239990234375, -0.025146484375, -0.029571533203125, -0.022491455078125, -0.02587890625, -0.02081298828125, -0.024688720703125, -0.026885986328125, -0.026214599609375, -0.025482177734375, -0.027374267578125, -0.03387451171875, -0.03570556640625, -0.0379638671875, -0.03662109375, -0.034637451171875, -0.03826904296875, -0.0408935546875, -0.037384033203125, -0.038177490234375, -0.039337158203125, -0.03564453125, -0.02972412109375, -0.02410888671875, -0.01873779296875, -0.02288818359375, -0.02679443359375, -0.03839111328125, -0.0316162109375, -0.029449462890625, -0.02972412109375, -0.03564453125, -0.034332275390625, -0.038665771484375, -0.044525146484375, -0.040374755859375, -0.039031982421875, -0.03741455078125, -0.039703369140625, -0.0386962890625, -0.036834716796875, -0.03521728515625, -0.033905029296875, -0.02984619140625, -0.035430908203125, -0.032440185546875, -0.029022216796875, -0.024688720703125, -0.024139404296875, -0.027099609375, -0.027313232421875, -0.02496337890625, -0.02203369140625, -0.0244140625, -0.021240234375, -0.02392578125, -0.020782470703125, -0.01873779296875, -0.0208740234375, -0.0208740234375, -0.022491455078125, -0.01806640625, -0.0216064453125, -0.017181396484375, -0.01397705078125, -0.01556396484375, -0.009979248046875, -0.016693115234375, -0.01068115234375, -0.016754150390625, -0.01959228515625, -0.016143798828125, -0.02447509765625, -0.029266357421875, -0.026947021484375, -0.02496337890625, -0.0345458984375, -0.027618408203125, -0.0318603515625, -0.028656005859375, -0.02685546875, -0.025634765625, -0.02392578125, -0.026031494140625, -0.014617919921875, -0.018585205078125, -0.021697998046875, -0.019317626953125, -0.02044677734375, -0.0184326171875, -0.018951416015625, -0.022125244140625, -0.019073486328125, -0.02203369140625, -0.0224609375, -0.02166748046875, -0.019073486328125, -0.015411376953125, -0.016448974609375, -0.023834228515625, -0.021728515625, -0.016387939453125, -0.009490966796875, -0.012542724609375, -0.0169677734375, -0.017822265625, -0.02105712890625, -0.017913818359375, -0.016815185546875, -0.01983642578125, -0.0179443359375, -0.0123291015625, -0.01129150390625, -0.01324462890625, -0.015869140625, -0.01385498046875, -0.016387939453125, -0.015655517578125, -0.0181884765625, -0.017578125, -0.013092041015625, -0.008331298828125, -0.007781982421875, -0.00439453125, -0.007080078125, -0.010223388671875, -0.01239013671875, -0.014923095703125, -0.01080322265625, -0.001983642578125, -0.0074462890625, -0.017791748046875, -0.023040771484375, -0.02978515625, -0.0267333984375, -0.0224609375, -0.017120361328125, -0.024871826171875, -0.01788330078125, -0.012298583984375, -0.011566162109375, -0.00726318359375, -0.00457763671875, -0.00299072265625, 0.00146484375, -0.0037841796875, -0.008819580078125, -0.0076904296875, -0.006256103515625, 0.001373291015625, -0.001708984375, -0.00335693359375, 0.001953125, 0.005859375, 0.00396728515625, 0.007110595703125, 0.011993408203125, 0.005828857421875, 0.00677490234375, 0.000244140625, 0.008575439453125, 0.0098876953125, 0.003875732421875, 0.0067138671875, 0.000946044921875, 0.00274658203125, 0.001800537109375, 0.00506591796875, 0.006072998046875, -0.006103515625, -0.00909423828125, -0.003936767578125, -0.001861572265625, -0.002777099609375, 0.001495361328125, 0.0006103515625, -0.003265380859375, -0.0003662109375, 0.00128173828125, 0.0010986328125, 0.002655029296875, -0.005615234375, -0.01275634765625, -0.00775146484375, -0.004913330078125, -0.004119873046875, -0.00506591796875, -9.1552734375e-05, 0.003204345703125, -0.002410888671875, -0.001800537109375, 0.001312255859375, 0.003173828125, -0.002899169921875, -0.004608154296875, 0.002593994140625, -0.002685546875, -0.00762939453125, -0.0028076171875, -0.006805419921875, -0.0146484375, -0.009979248046875, -0.00177001953125, 0.00286865234375, -0.0091552734375, -0.01495361328125, -0.01080322265625, -0.009368896484375, 0.0023193359375, -0.0010986328125, -0.001678466796875, -0.00177001953125, -0.006134033203125, -0.004730224609375, -0.00921630859375, -0.00909423828125, -0.0108642578125, -0.017181396484375, -0.015289306640625, -0.01458740234375, -0.013336181640625, -0.0057373046875, -0.004852294921875, -0.005645751953125, -0.0050048828125, -0.006500244140625, -0.00927734375, -0.012908935546875, -0.014404296875, -0.0155029296875, -0.0115966796875, -0.009796142578125, -0.01202392578125, -0.018157958984375, -0.021240234375, -0.015533447265625, -0.01629638671875, -0.01318359375, -0.015594482421875, -0.020721435546875, -0.017974853515625, -0.02056884765625, -0.02264404296875, -0.01654052734375, -0.01702880859375, -0.0146484375, -0.013275146484375, -0.023040771484375, -0.015960693359375, -0.013092041015625, -0.011077880859375, -0.009063720703125, -0.01727294921875, -0.018035888671875, -0.01580810546875, -0.011932373046875, -0.01287841796875, -0.003692626953125, -0.015167236328125, -0.014068603515625, -0.01666259765625, -0.0211181640625, -0.01812744140625, -0.013336181640625, -0.01519775390625, -0.0093994140625, -0.012847900390625, -0.0208740234375, -0.01300048828125, -0.006988525390625, -0.006072998046875, -0.011199951171875, -0.01263427734375, -0.01263427734375, -0.015625, -0.01055908203125, -0.00372314453125, -0.001312255859375, 0.001861572265625, -6.103515625e-05, -0.00311279296875, -0.001251220703125, -0.006500244140625, -0.00665283203125, 0.000823974609375, 0.001190185546875, 0.004486083984375, -0.004638671875, -0.00250244140625, -0.000518798828125, 0.001739501953125, 0.010955810546875, 0.00384521484375, -0.002349853515625, -0.00128173828125, -0.002227783203125, -0.005157470703125, -0.003204345703125, -0.00482177734375, -0.006072998046875, -0.001312255859375, -0.00018310546875, 0.0001220703125, -0.000274658203125, 0.003753662109375, 0.0103759765625, 0.009063720703125, 0.01324462890625, 0.019989013671875, 0.01324462890625, 0.015350341796875, 0.017791748046875, 0.019744873046875, 0.0157470703125, 0.007049560546875, 0.01263427734375, 0.0111083984375, 0.009002685546875, 0.01141357421875, 0.016632080078125, 0.012847900390625, 0.007568359375, 0.0042724609375, -0.00372314453125, -0.011383056640625, 0.00128173828125, 0.014312744140625, 0.016082763671875, 0.021697998046875, 0.020172119140625, 0.021575927734375, 0.02032470703125, 0.02215576171875, 0.02471923828125, 0.0302734375, 0.02752685546875, 0.02667236328125, 0.026580810546875, 0.0250244140625, 0.027557373046875, 0.020172119140625, 0.0247802734375, 0.02978515625, 0.030120849609375, 0.03131103515625, 0.031524658203125, 0.032257080078125, 0.0286865234375, 0.03033447265625, 0.0279541015625, 0.03582763671875, 0.036285400390625, 0.03515625, 0.028656005859375, 0.0311279296875, 0.033599853515625, 0.03582763671875, 0.028839111328125, 0.02947998046875, 0.0306396484375, 0.025146484375, 0.020843505859375, 0.027679443359375, 0.028045654296875, 0.02532958984375, 0.024017333984375, 0.02410888671875, 0.032073974609375, 0.018951416015625, 0.02801513671875, 0.0318603515625, 0.02587890625, 0.02825927734375, 0.025421142578125, 0.033203125, 0.03515625, 0.0362548828125, 0.030975341796875, 0.034332275390625, 0.02392578125, 0.027191162109375, 0.03472900390625, 0.03515625, 0.02813720703125, 0.0291748046875, 0.028717041015625, 0.027099609375, 0.02874755859375, 0.02203369140625, 0.019805908203125, 0.0179443359375, 0.0289306640625, 0.023773193359375, 0.017059326171875, 0.020904541015625, 0.0262451171875, 0.022979736328125, 0.021453857421875, 0.024017333984375, 0.02056884765625, 0.022430419921875, 0.02081298828125, 0.021759033203125, 0.026611328125, 0.033660888671875, 0.027374267578125, 0.02435302734375, 0.0185546875, 0.018096923828125, 0.023223876953125, 0.01654052734375, 0.015899658203125, 0.009490966796875, 0.00897216796875, 0.00933837890625, 0.013763427734375, 0.01470947265625, 0.021392822265625, 0.0238037109375, 0.022979736328125, 0.025665283203125, 0.0169677734375, 0.0174560546875, 0.015472412109375, 0.012786865234375, 0.011688232421875, 0.0103759765625, 0.00640869140625, 0.0113525390625, 0.0142822265625, 0.012603759765625, 0.0142822265625, 0.016815185546875, 0.020782470703125, 0.012237548828125, 0.008392333984375, 0.017578125, 0.019775390625, 0.026336669921875, 0.02557373046875, 0.019317626953125, 0.015380859375, 0.0196533203125, 0.01812744140625, 0.020050048828125, 0.015045166015625, 0.01416015625, 0.01129150390625, 0.00885009765625, 0.00799560546875, 0.01055908203125, 0.0107421875, 0.0164794921875, 0.0133056640625, 0.0064697265625, 0.0089111328125, 0.0069580078125, 0.0064697265625, 0.001220703125, -0.003082275390625, -0.0028076171875, -9.1552734375e-05, 0.00201416015625, -0.000946044921875, -0.001495361328125, 0.000579833984375, 0.003265380859375, 0.00390625, 0.005889892578125, 0.002685546875, -0.000732421875, 0.004058837890625, 0.0023193359375, 0.008544921875, 0.00250244140625, -0.000885009765625, -0.00244140625, -0.004608154296875, -0.002288818359375, -0.0050048828125, -0.000885009765625, -0.0013427734375, 0.001800537109375, 0.001678466796875, -0.005279541015625, 0.00506591796875, 0.002899169921875, 0.003662109375, 0.0087890625, 0.011474609375, 0.01422119140625, 0.01055908203125, 0.011444091796875, 0.012359619140625, 0.001190185546875, 0.0054931640625, 0.007598876953125, 0.01025390625, 0.01300048828125, 0.008575439453125, 0.007659912109375, 0.00897216796875, 0.014892578125, 0.01226806640625, 0.014434814453125, 0.022003173828125, 0.02056884765625, 0.022705078125, 0.02532958984375, 0.02154541015625, 0.02130126953125, 0.01788330078125, 0.016845703125, 0.018524169921875, 0.015167236328125, 0.01947021484375, 0.017578125, 0.01470947265625, 0.015533447265625, 0.015594482421875, 0.00836181640625, 0.0164794921875, 0.017608642578125, 0.012481689453125, 0.01287841796875, 0.01123046875, 0.010986328125, 0.01324462890625, 0.015655517578125, 0.01287841796875, 0.0107421875, 0.012908935546875, 0.00885009765625, 0.00201416015625, 0.008026123046875, 0.00994873046875, 0.011444091796875, 0.010894775390625, 0.01385498046875, 0.0174560546875, 0.014495849609375, 0.009246826171875, 0.00982666015625, 0.010406494140625, 0.015411376953125, 0.01507568359375, 0.0067138671875, 0.009521484375, 0.011322021484375, 0.00811767578125, -0.002410888671875, 0.00299072265625, -0.004852294921875, 0.0032958984375, 0.0032958984375, 6.103515625e-05, 0.00152587890625, 0.003082275390625, 0.011627197265625, 0.013458251953125, 0.01239013671875, 0.015777587890625, 0.023406982421875, 0.027923583984375, 0.024139404296875, 0.020721435546875, 0.022308349609375, 0.026519775390625, 0.019256591796875, 0.013214111328125, 0.0146484375, 0.015777587890625, 0.02001953125, 0.0150146484375, 0.01055908203125, 0.00897216796875, 0.00823974609375, 0.0013427734375, 0.005615234375, -0.00225830078125, -0.008087158203125, 0.005950927734375, 0.00762939453125, 0.003326416015625, 0.009002685546875, 0.006744384765625, 0.0101318359375, 0.00732421875, 0.004425048828125, 0.01068115234375, 0.001251220703125, 0.008758544921875, 0.018218994140625, 0.013885498046875, 0.014617919921875, 0.011383056640625, 0.01373291015625, 0.0115966796875, 0.00567626953125, 0.002716064453125, -0.000823974609375, 0.0025634765625, 0.0028076171875, 0.002044677734375, -0.000335693359375, 0.0029296875, 0.002655029296875, 0.002349853515625, 0.001678466796875, 0.00433349609375, 0.011871337890625, 0.006744384765625, 0.001129150390625, 0.000640869140625, -0.00042724609375, -0.007781982421875, -0.00433349609375, -0.002166748046875, 0.00189208984375, 0.000823974609375, -0.001922607421875, -0.000152587890625, -0.001007080078125, -0.005035400390625, -0.006439208984375, -0.00799560546875, -0.0150146484375, -0.017822265625, -0.02020263671875, -0.012542724609375, -0.01116943359375, -0.012298583984375, -0.017974853515625, -0.011810302734375, -0.009674072265625, -0.01446533203125, -0.0096435546875, -0.017852783203125, -0.0228271484375, -0.024505615234375, -0.022064208984375, -0.01568603515625, -0.01495361328125, -0.017242431640625, -0.014862060546875, -0.011871337890625, -0.009979248046875, -0.007965087890625, -0.007598876953125, -0.00628662109375, -0.009613037109375, -0.00982666015625, -0.0140380859375, -0.013275146484375, -0.016510009765625, -0.02313232421875, -0.019744873046875, -0.02117919921875, -0.024261474609375, -0.023406982421875, -0.025634765625, -0.026123046875, -0.029937744140625, -0.0272216796875, -0.025054931640625, -0.0198974609375, -0.020263671875, -0.022705078125, -0.0177001953125, -0.018585205078125, -0.020751953125, -0.01678466796875, -0.017181396484375, -0.016937255859375, -0.01995849609375, -0.014312744140625, -0.015350341796875, -0.016815185546875, -0.014129638671875, -0.02496337890625, -0.019317626953125, -0.023193359375, -0.017059326171875, -0.015533447265625, -0.020843505859375, -0.01788330078125, -0.021575927734375, -0.016876220703125, -0.0162353515625, -0.01556396484375, -0.02313232421875, -0.017822265625, -0.011871337890625, -0.0125732421875, -0.01348876953125, -0.014312744140625, -0.00909423828125, -0.009063720703125, -0.010345458984375, -0.00726318359375, -0.01397705078125, -0.009490966796875, -0.00982666015625, -0.007598876953125, -0.00421142578125, -0.00067138671875, 0.001953125, 0.001556396484375, 0.001220703125, -0.009185791015625, -0.013336181640625, -0.01556396484375, -0.01116943359375, -0.0096435546875, -0.010162353515625, -0.011749267578125, -0.012359619140625, -0.009124755859375, -0.009857177734375, -0.011474609375, -0.007568359375, -0.0068359375, -0.0062255859375, -0.00482177734375, -0.010467529296875, -0.0078125, -0.00750732421875, -0.01434326171875, -0.01361083984375, -0.0181884765625, -0.020782470703125, -0.007568359375, -0.006988525390625, -0.006622314453125, -0.001861572265625, -0.00128173828125, -0.0115966796875, -0.005401611328125, -0.004974365234375, -0.0084228515625, -0.011383056640625, -0.0118408203125, -0.008148193359375, -0.006256103515625, -0.001861572265625, 0.004302978515625, 0.004913330078125, 0.006195068359375, 0.00897216796875, 0.003753662109375, 0.00360107421875, -0.00201416015625, -0.001190185546875, -0.0030517578125, -0.0067138671875, -0.00469970703125, -0.005828857421875, -0.005645751953125, 0.001708984375, 0.002960205078125, 0.005767822265625, 0.001983642578125, 0.00048828125, -0.00103759765625, -0.001556396484375, 0.0, 0.007659912109375, 0.01202392578125, 0.010986328125, 0.0059814453125, 0.007354736328125, 0.01275634765625, 0.010009765625, 0.008880615234375, 0.008544921875, 0.007354736328125, 0.001800537109375, 0.00115966796875, -0.002410888671875, 0.009063720703125, 0.01190185546875, 0.012908935546875, 0.010650634765625, 0.004974365234375, 0.01251220703125, 0.012603759765625, 0.007110595703125, 0.00860595703125, 0.017303466796875, 0.01348876953125, 0.01556396484375, 0.0159912109375, 0.0147705078125, 0.01861572265625, 0.014068603515625, 0.0167236328125, 0.015533447265625, 0.0198974609375, 0.019866943359375, 0.015350341796875, 0.0079345703125, 0.0091552734375, 0.00921630859375, 0.011077880859375, 0.00738525390625, 0.008544921875, 0.01690673828125, 0.01513671875, 0.010009765625, 0.0107421875, 0.009674072265625, 0.0142822265625, 0.015899658203125, 0.012359619140625, 0.0203857421875, 0.02166748046875, 0.02032470703125, 0.02069091796875, 0.018280029296875, 0.010772705078125, 0.0057373046875, 0.013519287109375, 0.017242431640625, 0.011383056640625, 0.0142822265625, 0.013824462890625, 0.011962890625, 0.010284423828125, 0.0089111328125, 0.011993408203125, 0.0103759765625, -3.0517578125e-05, -0.00640869140625, -0.00506591796875, -0.00701904296875, -0.003143310546875, 0.0037841796875, 0.008209228515625, 0.00518798828125, 0.00506591796875, 0.006591796875, 0.00701904296875, 0.00567626953125, 0.011383056640625, 0.00543212890625, 0.001556396484375, 0.009185791015625, 0.00628662109375, 0.009521484375, 0.01324462890625, 0.0198974609375, 0.01837158203125, 0.017669677734375, 0.0103759765625, 0.013214111328125, 0.015594482421875, 0.014495849609375, 0.013092041015625, 0.010711669921875, 0.006195068359375, 0.0054931640625, 0.012969970703125, 0.01123046875, 0.017974853515625, 0.015106201171875, 0.011505126953125, 0.009307861328125, 0.024322509765625, 0.023284912109375, 0.01983642578125, 0.025726318359375, 0.030059814453125, 0.0242919921875, 0.02655029296875, 0.03326416015625, 0.023712158203125, 0.02374267578125, 0.022552490234375, 0.0157470703125, 0.020782470703125, 0.022064208984375, 0.022430419921875, 0.0272216796875, 0.02301025390625, 0.019744873046875, 0.018768310546875, 0.0240478515625, 0.029876708984375, 0.032196044921875, 0.030975341796875, 0.026458740234375, 0.025421142578125, 0.023529052734375, 0.024505615234375, 0.021697998046875, 0.018768310546875, 0.0145263671875, 0.01544189453125, 0.0244140625, 0.0198974609375, 0.017578125, 0.021148681640625, 0.01885986328125, 0.0191650390625, 0.018890380859375, 0.02740478515625, 0.018646240234375, 0.02069091796875, 0.025787353515625, 0.02423095703125, 0.0245361328125, 0.022796630859375, 0.01898193359375, 0.01727294921875, 0.021514892578125, 0.014739990234375, 0.01812744140625, 0.023651123046875, 0.020263671875, 0.01995849609375, 0.01971435546875, 0.021331787109375, 0.013336181640625, 0.01605224609375, 0.020111083984375, 0.0228271484375, 0.01959228515625, 0.0181884765625, 0.02130126953125, 0.00885009765625, 0.0120849609375, 0.012786865234375, 0.01593017578125, 0.021728515625, 0.021636962890625, 0.02227783203125, 0.017791748046875, 0.01885986328125, 0.025177001953125, 0.027557373046875, 0.019287109375, 0.01025390625, 0.01348876953125, 0.014129638671875, 0.02435302734375, 0.026336669921875, 0.02685546875, 0.0263671875, 0.029052734375, 0.03204345703125, 0.026580810546875, 0.033050537109375, 0.03021240234375, 0.02557373046875, 0.02392578125, 0.027801513671875, 0.0362548828125, 0.036041259765625, 0.03271484375, 0.03167724609375, 0.0325927734375, 0.038818359375, 0.036163330078125, 0.037017822265625, 0.030364990234375, 0.02996826171875, 0.029754638671875, 0.02813720703125, 0.021087646484375, 0.02264404296875, 0.020782470703125, 0.02197265625, 0.026580810546875, 0.020111083984375, 0.023834228515625, 0.02264404296875, 0.018157958984375, 0.026123046875, 0.027130126953125, 0.027618408203125, 0.031829833984375, 0.030487060546875, 0.027587890625, 0.025115966796875, 0.02667236328125, 0.0299072265625, 0.030426025390625, 0.0299072265625, 0.033599853515625, 0.035491943359375, 0.0390625, 0.035369873046875, 0.029266357421875, 0.022247314453125, 0.029083251953125, 0.022186279296875, 0.017181396484375, 0.02008056640625, 0.02447509765625, 0.027984619140625, 0.020782470703125, 0.0203857421875, 0.02197265625, 0.02520751953125, 0.018524169921875, 0.01922607421875, 0.02557373046875, 0.020599365234375, 0.025421142578125, 0.02606201171875, 0.026885986328125, 0.025970458984375, 0.0262451171875, 0.024200439453125, 0.0257568359375, 0.024078369140625, 0.02227783203125, 0.027923583984375, 0.0250244140625, 0.01995849609375, 0.022369384765625, 0.020538330078125, 0.021026611328125, 0.02734375, 0.0316162109375, 0.0347900390625, 0.0272216796875, 0.03057861328125, 0.034454345703125, 0.0289306640625, 0.035491943359375, 0.033538818359375, 0.023651123046875, 0.025848388671875, 0.0223388671875, 0.018646240234375, 0.01934814453125, 0.02130126953125, 0.01800537109375, 0.01824951171875, 0.01837158203125, 0.017242431640625, 0.021148681640625, 0.02520751953125, 0.02197265625, 0.021270751953125, 0.01971435546875, 0.0244140625, 0.02313232421875, 0.0244140625, 0.0272216796875, 0.0302734375, 0.023895263671875, 0.027374267578125, 0.031097412109375, 0.0198974609375, 0.0228271484375, 0.0255126953125, 0.026031494140625, 0.025299072265625, 0.030242919921875, 0.030487060546875, 0.029571533203125, 0.02880859375, 0.02398681640625, 0.029266357421875, 0.02618408203125, 0.026947021484375, 0.022216796875, 0.022247314453125, 0.022552490234375, 0.014373779296875, 0.011444091796875, 0.011444091796875, 0.012115478515625, 0.00823974609375, 0.01446533203125, 0.008636474609375, 0.00726318359375, 0.007720947265625, 0.010406494140625, 0.008758544921875, 0.00848388671875, 0.01226806640625, 0.009368896484375, 0.00732421875, -0.000823974609375, 0.00152587890625, 0.003631591796875, 0.00640869140625, 0.015655517578125, 0.0234375, 0.015960693359375, 0.010955810546875, 0.01055908203125, 0.009185791015625, 0.00994873046875, 0.016632080078125, 0.01751708984375, 0.015411376953125, 0.0157470703125, 0.0189208984375, 0.015167236328125, 0.009735107421875, 0.019439697265625, 0.024169921875, 0.02508544921875, 0.022308349609375, 0.020111083984375, 0.02056884765625, 0.018035888671875, 0.02093505859375, 0.018280029296875, 0.0152587890625, 0.0185546875, 0.01220703125, 0.01251220703125, 0.01544189453125, 0.01629638671875, 0.017120361328125, 0.01385498046875, 0.020416259765625, 0.017181396484375, 0.015960693359375, 0.01318359375, 0.009796142578125, 0.008148193359375, 0.01165771484375, 0.014892578125, 0.01531982421875, 0.013275146484375, 0.01507568359375, 0.0140380859375, 0.011993408203125, 0.0147705078125, 0.017547607421875, 0.013702392578125, 0.014678955078125, 0.014404296875, 0.0152587890625, 0.0140380859375, 0.01116943359375, 0.012176513671875, 0.009674072265625, 0.013153076171875, 0.013397216796875, 0.005462646484375, 0.011749267578125, 0.016021728515625, 0.010101318359375, 0.008819580078125, -0.000396728515625, 0.004852294921875, 0.000457763671875, 0.002838134765625, 0.0035400390625, -0.003662109375, 0.005950927734375, 0.00018310546875, 0.0047607421875, 0.0089111328125, 0.010345458984375, 0.005645751953125, 0.00897216796875, 0.009552001953125, 0.014862060546875, 0.012420654296875, 0.00762939453125, 0.009918212890625, 0.01318359375, 0.013824462890625, 0.01019287109375, 0.01519775390625, 0.018829345703125, 0.020782470703125, 0.022491455078125, 0.02142333984375, 0.01995849609375, 0.013580322265625, 0.01446533203125, 0.0179443359375, 0.012298583984375, 0.014556884765625, 0.01953125, 0.015777587890625, 0.017059326171875, 0.01171875, 0.01025390625, 0.020660400390625, 0.0185546875, 0.02239990234375, 0.026336669921875, 0.019989013671875, 0.01690673828125, 0.01507568359375, 0.0186767578125, 0.014434814453125, 0.01007080078125, 0.01788330078125, 0.016387939453125, 0.018280029296875, 0.016143798828125, 0.01678466796875, 0.012939453125, 0.014251708984375, 0.014923095703125, 0.01190185546875, 0.009674072265625, 0.014251708984375, 0.015106201171875, 0.008392333984375, 0.008544921875, 0.008514404296875, 0.011932373046875, 0.0032958984375, 0.002655029296875, 0.008544921875, 0.006622314453125, 0.012176513671875, 0.00640869140625, 0.008026123046875, 0.0126953125, 0.01043701171875, 0.003570556640625, 0.000457763671875, 0.001495361328125, 0.001190185546875, 0.0052490234375, 0.007659912109375, 0.00634765625, 0.003997802734375, 0.004150390625, 0.00885009765625, 0.00103759765625, 0.003936767578125, 0.00653076171875, 0.0006103515625, -0.000213623046875, 0.000579833984375, -0.001922607421875, 0.00189208984375, 0.002044677734375, 0.00689697265625, 0.005950927734375, 0.008514404296875, 0.010772705078125, 0.00347900390625, 0.008026123046875, 0.005218505859375, 0.005218505859375, 0.004669189453125, 0.011871337890625, 0.01348876953125, 0.015655517578125, 0.010223388671875, 0.0086669921875, 0.0128173828125, 0.0155029296875, 0.022369384765625, 0.018524169921875]
  out "FrameCount":i32 caption="Frame Count"
  out "SkippedFrames":i32 caption="Skipped Frames"
  out "AVIImage":T10(plugin-control)
  out "PupilClust":T11
  in  "Finished":bool
  in  "Database":T12={"ExperimentDate"=timestamp(0 s since 1904-01-01), "ImplantDate"=timestamp(3586535987.288034 s since 1904-01-01), "CerebusFolder"="", "Experimenter"="", "PatientNumber"="", "DominantHand"="", "DeviceType"="", "DeviceSerial"="", "DeviceHemisphere"="", "DeviceRegion"="", "TaskType"="", "TaskComments"="", "RecordingComments"="", "GeneralObservations"=""}
  in  "RecordSel":string(combo)
  in  "Comment":string caption="Realtime Comment"
  in  "SendComment":bool
  in  "CognitiveLoad":T13={"EEGTrigger"=FALSE, "ConnectECG"=FALSE, "TriggerECGwithTargets"=FALSE, "SecondaryTask"=FALSE, "MinTimeBetweenStimuli"=2000.0, "VariableTimeBetweenStimuli"=2000.0, "StimulusDuration"=1000.0}
  out "EventParamsFID":refnum<file>
  out "SelKin":cluster{"CurIdx":dbl, dbl, "RasterOut":dbl[]}[](graph)
  out "SelRate":cluster{"CurIdx":dbl, dbl, "RasterOut":dbl[]}[](graph)
  out "SelElect":u32=1
  out "EMGHMIdx":i32[](array[numeric])=[1, 2, 3, 4, 5, 6, 7, 8, 9, 10, 11, 12, 13, 14, 15, 16, 17, 18, 19, 20, 21, 22, 23, 24, 25, 26, 27, 28, 29, 30, 31, 32, 33, 34, 35, 36, 37, 38, 39, 40, 41, 42, 43, 44, 45, 46, 47, 48, 49, 50, 51, 52, 53, 54, 55, 56, 57, 58, 59, 60, 61, 62, 63, 64, 65, 66, 67, 68, 69, 70, 71, 72, 73, 74, 75, 76, 77, 78, 79, 80]
  out "EMGPos":T14={"[0]"=837, "[1]"=86, "[2]"=309, "[3]"=244}
  out "EMGHM":picture
  out "UlnarHM":picture
  out "MedianHM":picture
  out "TargDist":dbl[](array[numeric])
  out "FileIO":T15(ring)
  out "XMLFile":path=path "C:/Users/Administrator/Code/General/MSMS/Scenarios/MaleRight/Model/Prostheses/prosthesis.xml"
  out "Status":enum16{"In", "Out"}(ring)=enum."Out"
  out "BaseCnt2":u64
  in  "PltMode":enum16{"Rate", "Corr"}(ring)
  out "PrevIdx":dbl
  out "SubCase":i32=1
  in  "HoldCorr":bool
  in  "ResetCorr":bool
  out "UlnarPos":T14={"[0]"=521, "[1]"=86, "[2]"=309, "[3]"=244}
  out "TrialArray":string[](array[string])
  out "DataPath":path=path "D:/20150605-152610"
  out "Tracking":bool
  out "TrialTime (ms)":dbl=3000.0
  out "TargCnt":u64
  out "StimArray":dbl[](array[numeric])
  out "UEAHMIdx":i32[](array[numeric])=[10, 20, 30, 40, 50, 60, 70, 80, 90, 100, 9, 19, 29, 39, 49, 59, 69, 79, 89, 99, 8, 18, 28, 38, 48, 58, 68, 78, 88, 98, 7, 17, 27, 37, 47, 57, 67, 77, 87, 97, 6, 16, 26, 36, 46, 56, 66, 76, 86, 96, 5, 15, 25, 35, 45, 55, 65, 75, 85, 95, 4, 14, 24, 34, 44, 54, 64, 74, 84, 94, 3, 13, 23, 33, 43, 53, 63, 73, 83, 93, 2, 12, 22, 32, 42, 52, 62, 72, 82, 92, 1, 11, 21, 31, 41, 51, 61, 71, 81, 91]
  in  "HMSize":cluster{"NumCol":dbl, "NumRows":dbl}={"NumCol"=10.0, "NumRows"=10.0}
  out "MedianPos":T14={"[0]"=204, "[1]"=86, "[2]"=309, "[3]"=244}
